vi "Prompted Inputs Updater.vi"() -> ()   [LabVIEW 2011]
uses:
  <userlib>/_OpenG.lib/file/file.llb/Convert File Extension (Path)__ogtk.vi
  <userlib>/_OpenG.lib/file/file.llb/Valid Path - Traditional__ogtk.vi
  <vilib>/addons/internet/http/config.llb/HTTP SRM.vi
  SI.LIB/OGAB Version.ctl
panel:
  out "Status":string
  in  "spartan install path":path=path "C:/Development/Spartan"
  out "Database Operation":string
  out "Spartan Install Path":path
  out "ver":string
  in  "Version":T1 {"Build Date/Time" format="%<%X\n%x>T"}
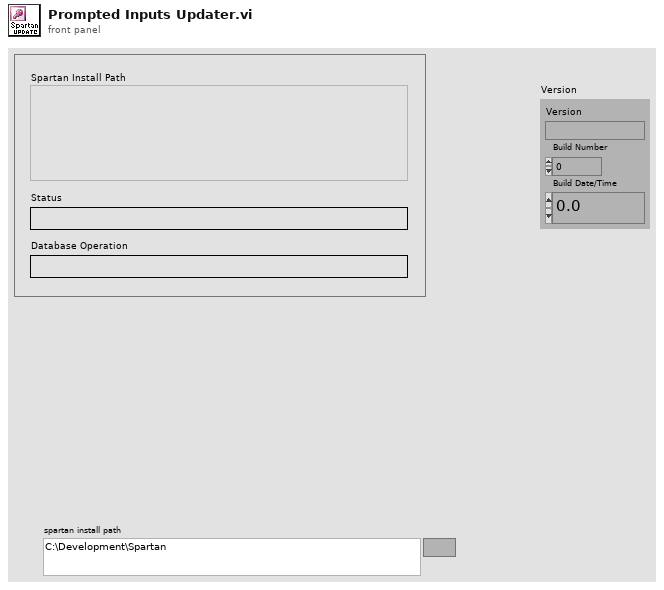
[diagram p1: front panel]
types:
  T1 = typedef "OGAB Version.ctl" = cluster{"Version":string, "Build Number":u32, "Build Date/Time":dbl}
  T2 = typedef "Connection Refnum.ctl" = cluster{"Environment Handle":i32, "Connection Handle":i32}
  T3 = typedef "Step Record.ctl" = cluster{"ixStep":i32, "sxSequenceId":string, "sxTestId":string, "iIndex":i32, "iRepeat":i32, "iQuickMode":i32, "sTag":string, "sDatasheetsCSV":string, "bConfiguration":string}
  T4 = typedef "PI Test Parameters.ctl" = cluster{"Measurement":T5, "Limit":T6}
  T5 = typedef "PI Measurement Cluster.ctl" = cluster{"sxFieldId":string, "sValue":string, "nDataType":enum16{"Scalar", "Enumeration"}, "sUnits":string, "sDisplayName":string}
  T6 = typedef "PI Limit Parameters.ctl" = cluster{"Limits On":bool, "Limits":T7[]}
  T7 = typedef "PI Limit Definition.ctl" = cluster{"nComparison":T8, "sValue":string}
  T8 = typedef "PI Limit Comparison.ctl" = enum16{">", ">=", "<", "<=", "<>", "="}
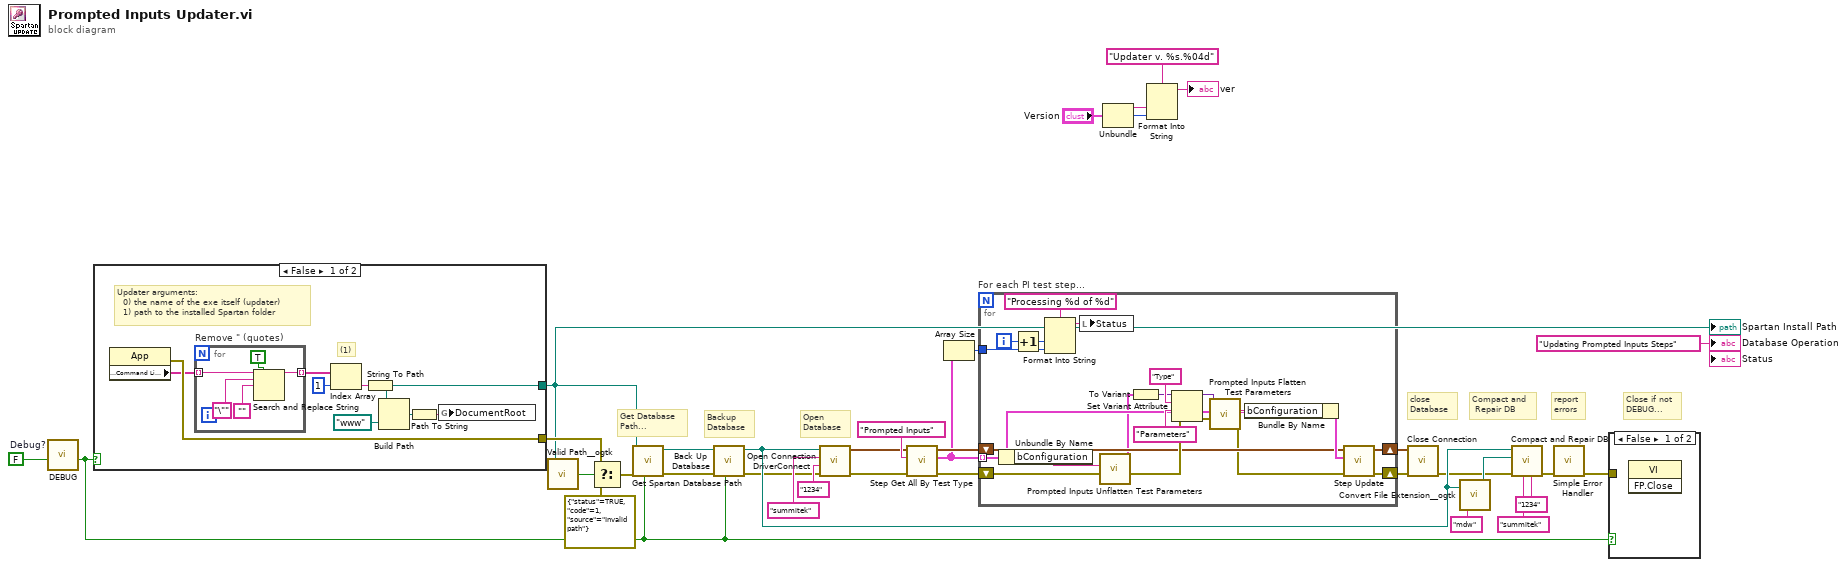
[diagram p0: block diagram]
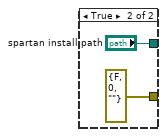
[diagram p3: hidden frame]
diagram:
  w29 = FALSE  # Debug?
  # "Backup\nDatabase"
  # "close\nDatabase"
  # "Compact and\n Repair DB"
  # "Open\nDatabase"
  # "Get Database\nPath..."
  # "report\nerrors"
  # "Close if not\nDEBUG..."
  n1 = call "DEBUG.vi"("Dev DEBUG? (f)"=w29) -> ("DEBUG?"=w22:bool)  [unwired: 1 in, 5 out]
  n2 = case shown="False" w22 {
    tunnel: [w38 "spartan install path"] -> w23
    tunnel: [w44 errorcluster {"status"=FALSE, "code"=0, "source"=""} ("error out")] -> w27
    frame False {
      # "(1)"
      # "Updater arguments:\n  0) the name of the exe itself (updater)\n  1) path to the installed Spartan folder"
      n3 = property class="App"() -> (error out=w44:errorcluster, "Application:Command Line Arguments"=w43:string[])  [unwired: 2 in, 1 out]
      n4 = for "Remove \" (quotes)" {
        tunnel: w43 -> [w47] mode=indexing
        tunnel: [w46] -> w41 mode=indexing
        n5 = Search and Replace String(replace all?=TRUE, input string=w47, search string="\"", replace string="") -> (result string=w46:string)  [unwired: 1 in, 6 out]
      }
      n6 = Index Array(array=w41, index=1) -> (element=w40:string)
      n7 = String To Path(string=w40) -> (path=w38:path)
      n8 = Build Path(base path=w38, name or relative path=path "www" ("stripped path")) -> (appended path=w37:path)
      n9 = Path To String(path=w37) -> (string=w36:string)
      n10 = global write "HTTP SRM.vi" "DocumentRoot"(w36) -> ()
    }
    frame True {
    }
  }
  "Spartan Install Path" <- w23
  n11 = call-poly <userlib>:"Valid Path__ogtk.vi"("path"=w23) -> ("valid"=w28:bool)
  n12 = Select(t=w27, s=w28, f=errorcluster {"status"=TRUE, "code"=1, "source"="Invalid path"} ("error out")) -> (s? t:f=w21:errorcluster)
  n13 = call "Get Spartan Database Path.vi"("DEBUG? (f)"=w22, "error in (no error)"=w21, "Spartan Install Path (empty)"=w23) -> ("error out"=w1:errorcluster, "Spartan Database Path"=w24:path)  [unwired: 7 out]
  n14 = call "Back Up Database.vi"("DEBUG? (f)"=w22, "error in (no error)"=w1, "Database Path (empty)"=w24) -> ("error out"=w12:errorcluster, "dup Database Path"=w13:path)  [unwired: 7 out]
  n15 = call "Open Connection DriverConnect.vi"("error in (no error)"=w12, "Password (\"\")"="1234" ("Username (\"\")"), "Username (\"\")"="summitek" ("Username (\"\")"), "ODBC Database (\"\")"=w13) -> ("error out"=w8:errorcluster, "Connection Refnum"=w7:T2)  [unwired: 3 out]
  n16 = call "Step Get All By Test Type.vi"("error in (no error)"=w8, "sxTestId (\"\")"="Prompted Inputs" ("Test Type"), "Connection Refnum"=w7) -> ("error out"=w6:errorcluster, "Sequence Steps"=w3:T3[], "Connection Refnum"=w5:T2)  [unwired: 1 in, 5 out]
  n17 = Array Size(array=w3) -> (size(s)=w2:i32)
  n18 = for "For each PI test step..." {
    shift-right: [w62] -> w11
    shift-left: w6 -> [w72]
    tunnel: w3 -> [w59] mode=indexing
    shift-right: [w60] -> w4
    shift-left: w5 -> [w61]
    tunnel: w2 -> [w52]
    i -> [w54]
    n19 = Unbundle By Name(w59) -> ("bConfiguration"=w71:string)
    n20 = Increment(x=w54) -> (x+1=w53:i32)
    n21 = Format Into String(format string="Processing %d of %d", w53, w52) -> (resulting string=w56:string)  [unwired: 2 in, 1 out]
    n22 = local write "Status"(w56) -> ()
    n23 = call "Prompted Inputs Unflatten Test Parameters.vi"("error in (no error)"=w72, "Parameter String"=w71) -> ("error out"=w63:errorcluster, "Prompted Inputs Test Parameters"=w57:T4)  [unwired: 8 out]
    n24 = To Variant(anything=w57) -> (Variant=w64:variant)
    n25 = Set Variant Attribute(Variant=w64, name="Type", value="Parameters" ("name"), error in=w63) -> (Variant out=w68:variant, error out=w65:errorcluster)  [unwired: 1 out]
    n26 = call "Prompted Inputs Flatten Test Parameters.vi"("error in (no error)"=w65, "Parameter Variant"=w68) -> ("error out"=w58:errorcluster, "Parameter String"=w69:string)  [unwired: 8 out]
    n27 = Bundle By Name(cluster=w59, "bConfiguration"=w69) -> (w70:T3)
    n28 = call "Step Update.vi"("error in (no error)"=w58, "Step Record (empty)"=w70, "Connection Refnum"=w61) -> ("error out"=w62:errorcluster, "Connection Refnum"=w60:T2)  [unwired: 7 out]
  }
  n29 = Unbundle("Version") -> ("Version"=w32:string, "Build Number"=w33:u32)  [unwired: 1 out]
  n30 = Format Into String(format string="Updater v. %s.%04d", w32, w33) -> (resulting string=→"ver":string)  [unwired: 2 in, 1 out]
  n31 = call "Close Connection.vi"("error in (no error)"=w11, "Connection Refnum"=w4) -> ("error out"=w10:errorcluster)  [unwired: 5 out]
  n32 = call-poly <userlib>:"Convert File Extension__ogtk.vi"("new ending (none)"="mdw", "file name"=w13) -> ("new filename"=w18:path)  [unwired: 1 out]
  n33 = call "Compact and Repair DB.vi"("password (\"\")"="1234" ("password (\"\")"), "username (\"\")"="summitek" ("username (\"\")"), "error in (no error)"=w10, "Workgroup DB (none)"=w18, "Database Path (empty)"=w13) -> ("error out"=w34:errorcluster)  [unwired: 6 out]
  n34 = call <vilib>:"Simple Error Handler.vi"("error in (no error)"=w34) -> ("error out"=w35:errorcluster)  [unwired: 1 in, 7 out]
  n35 = case shown="False" w22 {
    tunnel: w35 -> [_ _]
    frame False {
      n36 = invoke class="VI" method="FP.Close"() -> ()  [unwired: 3 in, 3 out]
    }
    frame True {
    }
  }
  "Database Operation" <- "Updating Prompted Inputs Steps"
